vi "EMG_SignalGenerate.vi"(11 "EMG_Channels_N":i32) -> (7 "Array":dbl[](array[numeric]))   [LabVIEW 2025]
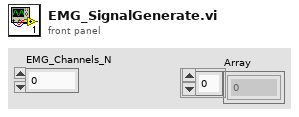
[diagram p1: front panel]
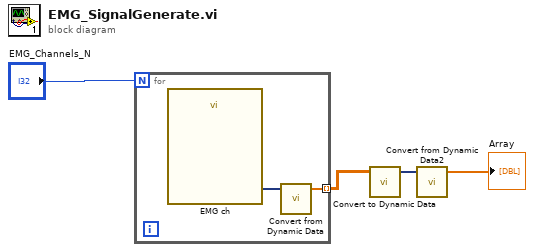
[diagram p0: block diagram]
diagram:
  n1 = for {
    N: "EMG_Channels_N" -> [_]
    tunnel: [w5] -> w4 mode=indexing
    n2 = call "EMG ch"() -> ("Sine with Gaussian Noise"=w6:dynamicdata)  [unwired: 14 in, 1 out]
    n3 = call "Convert from Dynamic Data"("Dynamic Data Type"=w6) -> ("Array"=w5:dbl[])  [unwired: 3 in]
  }
  n4 = call "Convert to Dynamic Data"("2D Array"=w4) -> ("Dynamic Data Type"=w3:dynamicdata)  [unwired: 3 in]
  n5 = call "Convert from Dynamic Data2"("Dynamic Data Type"=w3) -> ("Array"=→"Array":dbl[])  [unwired: 3 in]
